vi "Voltage - Function Generation.vi"() -> ()   [LabVIEW 2022 SP3]
doc: "This example demonstrates how to generate a continuous sine, triangle, square, or sawtooth waveform.\n\nFor instructions on how to connect your signals to the DAQ device, refer to your device documentation."
uses:
  <vilib>/Utility/error.llb/DialogType.ctl
  <vilib>/DAQmx/create/channels.llb/DAQmx Create Channel (AO-FuncGen).vi
panel:
  in  "Waveform Type":i32(ring)=14751 items=["Sine"=14751, "Triangle"=14752, "Square"=14753, "Sawtooth"=14754]
  in  "Frequency (Hz)":dbl=1000.0 format="%.2f"
  in  "Amplitude (V)":dbl=5.0 format="%.2f"
  in  "Offset (V)":dbl format="%.2f"
  in  "Stop":bool
  in  "Physical Channel(s)":tag="Dev1/ao0"
  # "Channel Settings"
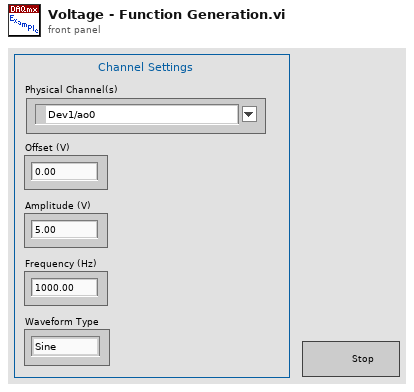
[diagram p1: front panel]
types:
  T1 = typedef "DialogType.ctl" = u16
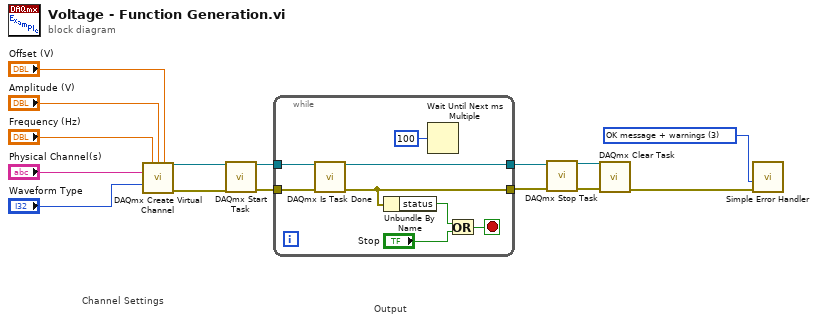
[diagram p0: block diagram]
diagram:
  w7 = T1 3 items=["no dialog", "OK message", "continue or stop message", "OK message + warnings", "continue/stop + warnings"] ("type of dialog (OK msg:1)")
  # "Output"
  # "Channel Settings"
  n1 = call-poly <vilib>:"DAQmx Create Virtual Channel.vi"("frequency"="Frequency (Hz)", "amplitude"="Amplitude (V)", "offset"="Offset (V)", "physical channels"="Physical Channel(s)", "type"="Waveform Type") -> ("task out"=w5:refnum<k21>, "error out"=w6:errorcluster)  [unwired: 9 in]
  n2 = call <vilib>:"DAQmx Start Task.vi"("task/channels in"=w5, "error in"=w6) -> ("task out"=w15:refnum<k21>, "error out"=w14:errorcluster)  [unwired: 12 in]
  n3 = while {
    tunnel: w15 -> [w23]
    tunnel: w14 -> [w22]
    tunnel: [w19] -> w8
    tunnel: [w20] -> w9
    stop <- w21 stop-if-true
    n4 = call <vilib>:"DAQmx Is Task Done.vi"("task/channels in"=w23, "error in"=w22) -> ("task out"=w20:refnum<k21>, "error out"=w19:errorcluster)  [unwired: 11 in, 1 out]
    n5 = Unbundle By Name(w19) -> ("status"=w18:bool)
    n6 = Wait Until Next ms Multiple(millisecond multiple=u32 100) -> ()  [unwired: 1 out]
    n7 = Or(x=w18, y="Stop") -> (x .or. y?=w21:bool)
  }
  n8 = call <vilib>:"DAQmx Stop Task.vi"("task/channels in"=w9, "error in"=w8) -> ("task out"=w11:refnum<k21>, "error out"=w10:errorcluster)  [unwired: 12 in]
  n9 = call <vilib>:"DAQmx Clear Task.vi"("task in"=w11, "error in"=w10) -> ("error out"=w13:errorcluster)  [unwired: 13 in]
  n10 = call <vilib>:"Simple Error Handler.vi"("type of dialog (OK msg:1)"=w7, "error in (no error)"=w13) -> ()  [unwired: 3 in, 5 out]
